vi "HB_GetFirmwareVersion.vi"(8 "error in (no error)":errorcluster, 11 "HBDeviceRef":T1) -> (0 "error IO":errorcluster, 1 "Firmware Version":string, 2 "Version Byte Array":u8[](array[numeric]), 3 "HBDeviceRef":T1)   [LabVIEW 2016]
uses:
  <vilib>/Rock Robotics/WPI/SerialPort/WPI_SerialPortRef.ctl
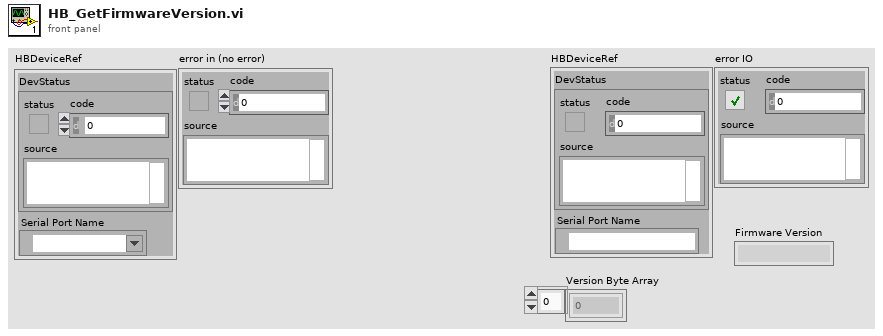
[diagram p1: front panel]
types:
  T1 = typedef "WPI_SerialPortRef.ctl" = cluster{"DevStatus":errorcluster, "Serial Port Name":refnum<visa-resource-name>}
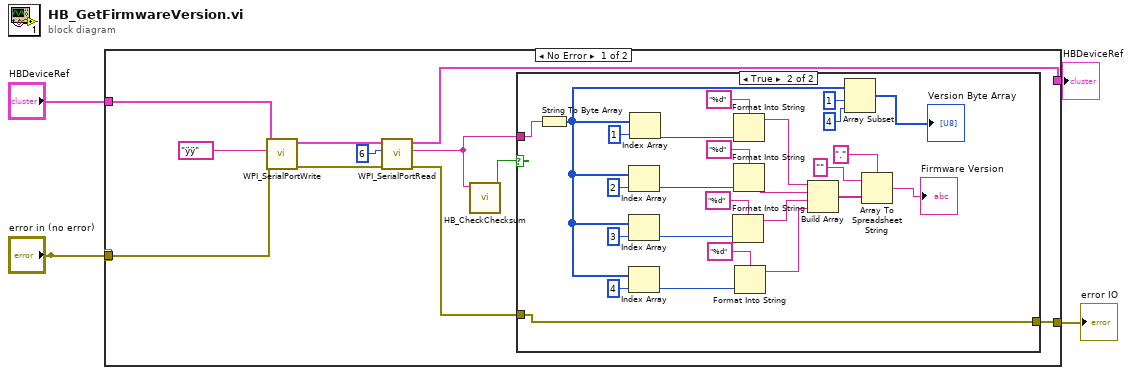
[diagram p0: block diagram]
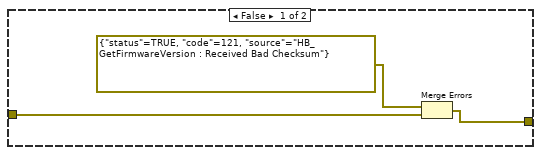
[diagram p2: hidden frame]
diagram:
  n1 = case shown="No Error" "error in (no error)" {
    selector: "error in (no error)" -> [_ w45]
    tunnel: "HBDeviceRef" -> [w12 w46]
    tunnel: "error in (no error)" -> [w11 _]
    tunnel: [w9 w46] -> w1
    tunnel: [w5 w45] -> w2
    frame No Error {
      n2 = call <vilib>:"WPI_SerialPortWrite.vi"("error in (no error)"=w11, "Buffer"="ÿÿ", "SerialPortRef"=w12) -> ("error out"=w13:errorcluster, "SerialPortRef"=w14:T1)  [unwired: 6 in, 1 out]
      n3 = call <vilib>:"WPI_SerialPortRead.vi"("error in (no error)"=w13, "Num Bytes to Read"=u32 6, "SerialPortRef"=w14) -> ("error out"=w6:errorcluster, "Buffer"=w7:string, "SerialPortRef"=w9:T1)  [unwired: 6 in]
      n4 = call <vilib>:"HB_CheckChecksum.vi"("String"=w7) -> ("Checksum Matches"=w8:bool)  [unwired: 9 in, 1 out]
      n5 = case shown="True" w8 {
        tunnel: w7 -> [_ w22]
        tunnel: w6 -> [w18 w21]
        tunnel: [w16 w21] -> w5
        frame False {
          n6 = Merge Errors(errorcluster {"status"=TRUE, "code"=121, "source"="HB_GetFirmwareVersion : Received Bad Checksum"} ("error out"), w18) -> (w16:errorcluster)
        }
        frame True {
          n7 = String To Byte Array(string=w22) -> (unsigned byte array=w26:u8[])
          n8 = Index Array(array=w26, index=2) -> (element=w35:u8)
          n9 = Index Array(array=w26, index=3) -> (element=w34:u8)
          n10 = Index Array(array=w26, index=4) -> (element=w33:u8)
          n11 = Index Array(array=w26, index=1) -> (element=w40:u8)
          n12 = Format Into String(format string="%d", w34) -> (resulting string=w30:string)  [unwired: 2 in, 1 out]
          n13 = Format Into String(format string="%d", w40) -> (resulting string=w32:string)  [unwired: 2 in, 1 out]
          n14 = Format Into String(format string="%d", w35) -> (resulting string=w31:string)  [unwired: 2 in, 1 out]
          n15 = Format Into String(format string="%d", w33) -> (resulting string=w29:string)  [unwired: 2 in, 1 out]
          n16 = Build Array(w32, w31, w30, w29) -> (w20:string[])
          n17 = Array Subset(array=w26, index=1, length=4) -> (→"Version Byte Array":u8[])
          n18 = Array To Spreadsheet String(delimiter (Tab)=".", array=w20, 3:"" ("format string")) -> (spreadsheet string=→"Firmware Version":string)
        }
      }
    }
    frame Error {
    }
  }
  "HBDeviceRef" <- w1
  "error IO" <- w2
